vi "Send.vi"(8 "error in (no error)":errorcluster, 10 "Message":refnum<class "MSG.lvclass">, 11 "Parallel Process in":refnum<class "Parallel Process.lvclass">) -> (0 "error out":errorcluster, 3 "Parallel Process out":refnum<class "Parallel Process.lvclass">)   [LabVIEW 2011, in "Messenging.lvlib" / "Parallel Process.lvclass"]
uses:
  Parallel Process.lvclass
  Interprocess Messenger/Messenger (Parent)/MGR.lvclass
  Interprocess Messenger/TextVarientMessage/MSG.lvclass
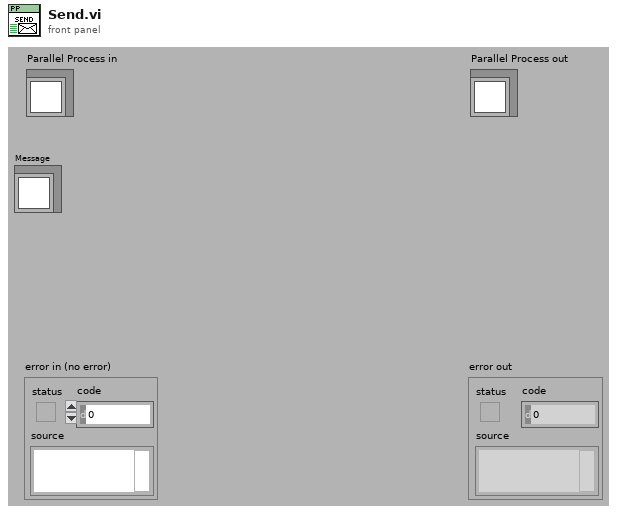
[diagram p1: front panel]
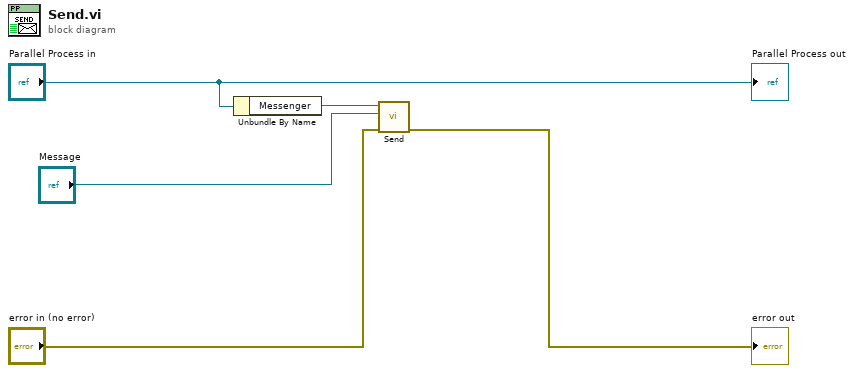
[diagram p0: block diagram]
diagram:
  n1 = Unbundle By Name("Parallel Process in") -> ("Messenger"=w1:refnum<class "MGR.lvclass">)
  n2 = call-dynamic "Send.vi"("error in (no error)"="error in (no error)", "Message"="Message", "MSR Parent in"=w1) -> ("error out"=→"error out":errorcluster)  [unwired: 8 out]
  "Parallel Process out" <- "Parallel Process in"
